vi "Four Bytes to Number.vi"(0 "VISA resource name":refnum<visa-resource-name>, 1 "Index 0 (3)":i8=3 min=3 max=25, 2 "Input Command Frame":string, 5 "Index 1 (4)":i8=4 min=3 max=25, 7 "Index 2 (5)":i8=5 min=3 max=25, 9 "Index 3 (6)":i8=6 min=3 max=25, 11 "error in (no error)":errorcluster, 13 "Decimal Offset (3)":i8=3 min=3 max=4) -> (4 "VISA resource name out":refnum<visa-resource-name>, 8 "Numerical Value":dbl format="%#.3g", 15 "error out":errorcluster)   [LabVIEW 2019, in "BK Precision 178XB Series.lvlib"]
doc: "This SubVI scans through <b>Input command frame</b> and takes four bytes out of the string selected by index 0, index 1, index 2, and index 3. Then, the bytes get arranged in little-endian format, converted from hexadecimal to integer, and formatted to a decimal value at the <b>Numerical Value</b> output. The <b>Decimal Offset</b> value is either 3 or 4. Use 3 if using this VI to read voltage, power, or resistance values. Use 4 to read current. Refer to Context Help of <b>Decimal Offset</b> for more details."
uses:
  BK Precision 178XB Series.lvlib
panel:
  # "(c) 2009 B&K PRECISION CORPORATION.  ALL RIGHTS RESERVED."
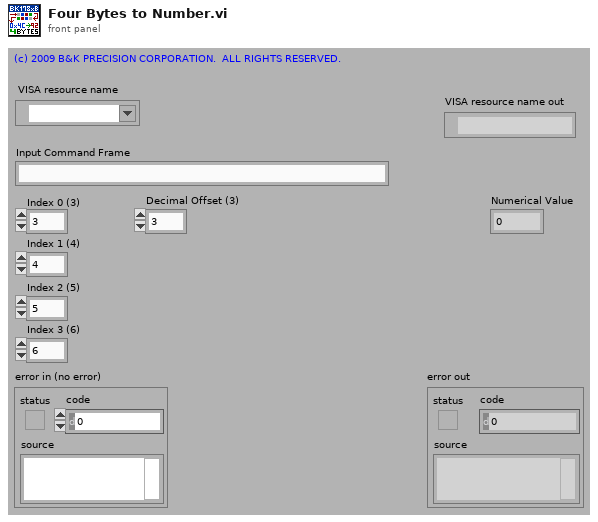
[diagram p1: front panel]
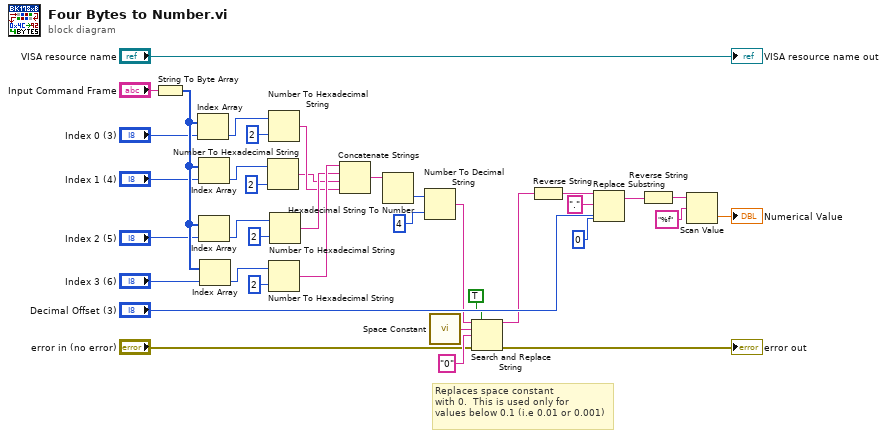
[diagram p0: block diagram]
diagram:
  # "Replaces space constant\nwith 0.  This is used only for\nvalues below 0.1 (i.e 0.01 or 0.001)"
  n1 = String To Byte Array(string="Input Command Frame") -> (unsigned byte array=w30:u8[])
  n2 = Index Array(array=w30, index="Index 0 (3)") -> (element=w32:u8)
  n3 = Index Array(array=w30, index="Index 1 (4)") -> (element=w18:u8)
  n4 = Index Array(array=w30, index="Index 2 (5)") -> (element=w33:u8)
  n5 = Index Array(array=w30, index="Index 3 (6)") -> (element=w34:u8)
  n6 = Number To Hexadecimal String(1:2, 2:w18) -> (0:w19:string)
  n7 = Number To Hexadecimal String(1:2, 2:w32) -> (0:w35:string)
  n8 = Number To Hexadecimal String(1:2, 2:w34) -> (0:w37:string)
  n9 = Number To Hexadecimal String(1:2, 2:w33) -> (0:w36:string)
  n10 = Concatenate Strings(w37, w36, w19, w35) -> (w9:string)
  n11 = Hexadecimal String To Number(string=w9) -> (number=w13:u32)  [unwired: 2 in, 1 out]
  n12 = Number To Decimal String(number=w13, width (-)=4 ("length (len. of substring)")) -> (decimal integer string=w8:string)
  n13 = call <vilib>:"Space Constant.vi"() -> ("String"=w7:string)
  n14 = Search and Replace String(replace all?=TRUE, input string=w8, search string=w7, replace string="0", error in="error in (no error)") -> (result string=w2:string, error out=→"error out":errorcluster)  [unwired: 3 in, 2 out]
  n15 = Reverse String(1:w2) -> (0:w12:string)
  n16 = Replace Substring(2:0 ("length (len. of substring)"), 3:"Decimal Offset (3)", 4:"." ("substring (\"\")"), 5:w12) -> (1:w11:string)  [unwired: 1 out]
  n17 = Reverse String(1:w11) -> (0:w22:string)
  n18 = Scan Value(string=w22, format string="%f") -> (value=→"Numerical Value":dbl)  [unwired: 1 in, 1 out]
  "VISA resource name out" <- "VISA resource name"
